vi "RotateMatrix.vi"(1 "gamma":dbl, 2 "beta":dbl, 3 "alpha":dbl) -> (0 "Rotate Matrix":T1)   [LabVIEW 2018]
uses:
  <vilib>/Analysis/Matrix/Datatypes/RealMatrix.ctl
  <vilib>/Analysis/Matrix/NI_Matrix.lvlib
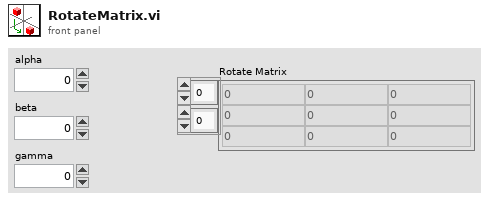
[diagram p1: front panel]
types:
  T1 = typedef "NI_Matrix.lvlib/RealMatrix.ctl" = dbl[][]
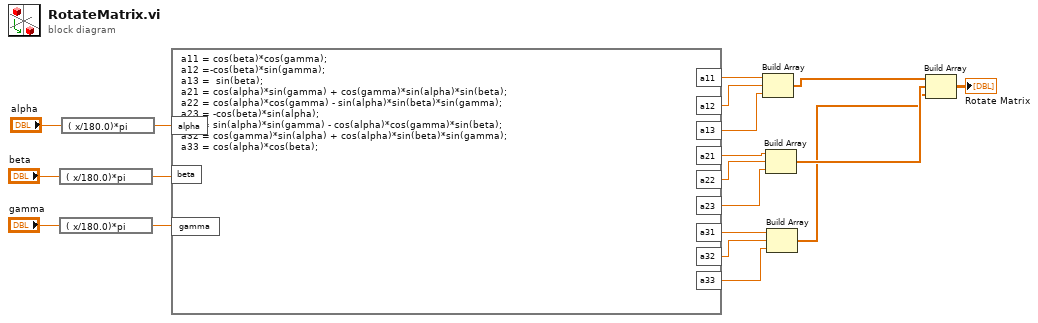
[diagram p0: block diagram]
diagram:
  n1 = expression code="( x/180.0)*pi"("beta") -> (w15:dbl)
  n2 = expression code="( x/180.0)*pi"("gamma") -> (w14:dbl)
  n3 = expression code="( x/180.0)*pi"("alpha") -> (w18:dbl)
  n4 = formula code="a11 = cos(beta)*cos(gamma);\na12 =-cos(beta)*sin(gamma);\na13 =  sin(beta);\na21 = cos(alpha)*sin(gamma) + cos(gamma)*sin(alpha)*sin(beta);\na22 = cos(alpha)*cos(gamma) - sin(alpha)*sin(beta)*sin(gamma);\na23 = -cos(beta)*sin(alpha);\na31 = sin(alpha)*sin(gamma) - cos(alpha)*cos(gamma)*sin(beta);\na32 = cos(gamma)*sin(alpha) + cos(alpha)*sin(beta)*sin(gamma);\na33 = cos(alpha)*cos(beta);"("alpha"=w18, "beta"=w15, "gamma"=w14) -> ("a11"=w13:dbl, "a12"=w12:dbl, "a13"=w11:dbl, "a21"=w10:dbl, "a22"=w9:dbl, "a23"=w8:dbl, "a31"=w7:dbl, "a32"=w6:dbl, "a33"=w5:dbl)
  n5 = Build Array(w13, w12, w11) -> (w4:dbl[])
  n6 = Build Array(w10, w9, w8) -> (w3:dbl[])
  n7 = Build Array(w7, w6, w5) -> (w2:dbl[])
  n8 = Build Array(w4, w3, w2) -> (→"Rotate Matrix":T1)
